vi "PDU Write Current.vi"(8 "error in (no error)":errorcluster, 10 "Current":dbl, 11 "Power Distribution in":refnum<class "Power Distribution.lvclass">) -> (0 "error out":errorcluster, 3 "Power Distribution out":refnum<class "Power Distribution.lvclass">)   [LabVIEW 2022 SP3, in "Power Distribution.lvclass"]
uses:
  Power Distribution.lvclass
  Power Distribution.lvclass/Power Distribution.ctl
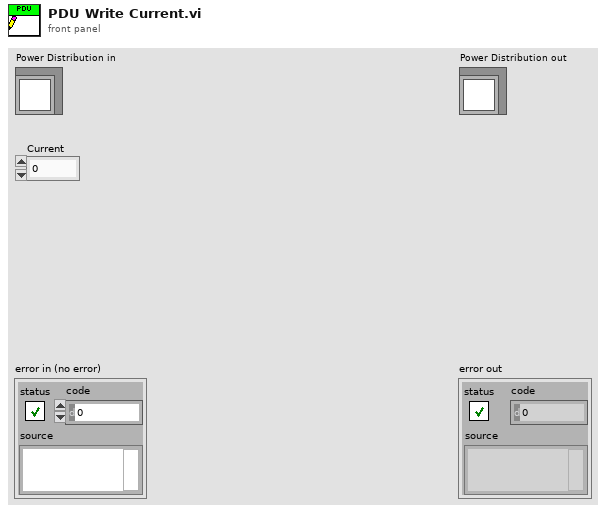
[diagram p1: front panel]
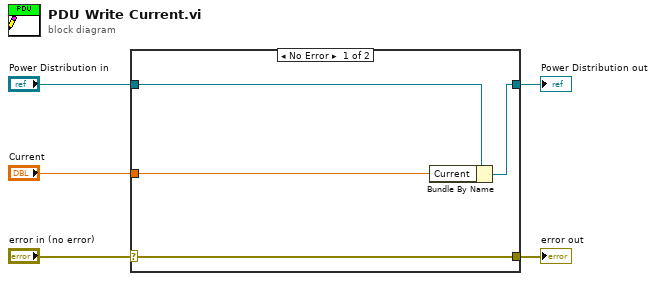
[diagram p0: block diagram]
diagram:
  n1 = case shown="No Error" "error in (no error)" {
    selector: "error in (no error)" -> [w9 w10]
    tunnel: [w9 w10] -> w4
    tunnel: [w7 w11] -> w2
    tunnel: "Power Distribution in" -> [w8 w11]
    tunnel: "Current" -> [w6 _]
    frame No Error {
      n2 = Bundle By Name(cluster=w8, "Current"=w6) -> (w7:refnum<class "Power Distribution.lvclass">)
    }
    frame Error {
    }
  }
  "error out" <- w4
  "Power Distribution out" <- w2
